vi "Create Value - Known Type.vi"(5 "JSON Compatible Type":T1=enum."Unknown", 7 "JSON Type":T2=enum."Unknown", 8 "error in (no error)":errorcluster, 10 "Value":variant) -> (0 "error out":errorcluster, 3 "JSON Tree":variant)   [LabVIEW 2013, in "i3-json.lvlib"]
uses:
  i3-json.lvlib
  JSON Types/JSON Type.ctl
  JSON Types/JSON Compatible Type.ctl
  JSON Types/JSON Variant Attribute.ctl
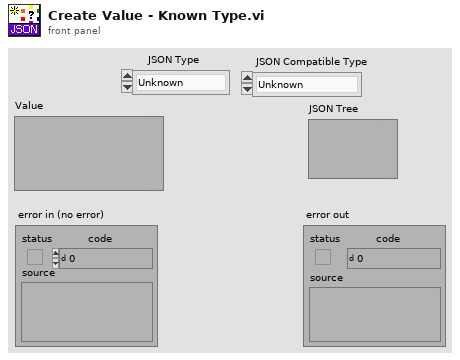
[diagram p1: front panel]
types:
  T1 = typedef "i3-json.lvlib/JSON Compatible Type.ctl" = enum16{"1D Double Array", "1D String Array", "1D Boolean Array", "Unknown"}
  T2 = typedef "i3-json.lvlib/JSON Type.ctl" = enum8{"JSON Compatible", "JSON Array", "JSON Object", "JSON Null", "Double", "String", "Boolean", "Unknown", "Data JSON string"}
  T3 = typedef "i3-json.lvlib/JSON Variant Attribute.ctl" = string
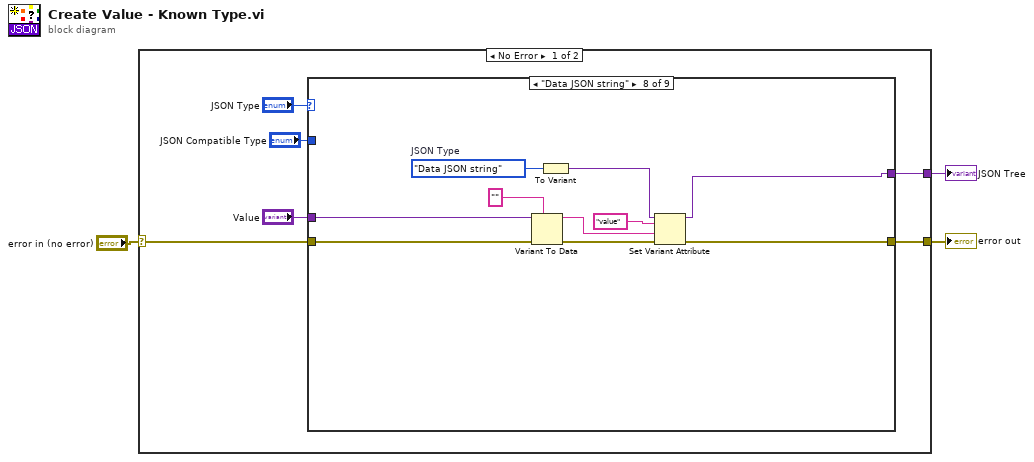
[diagram p0: block diagram]
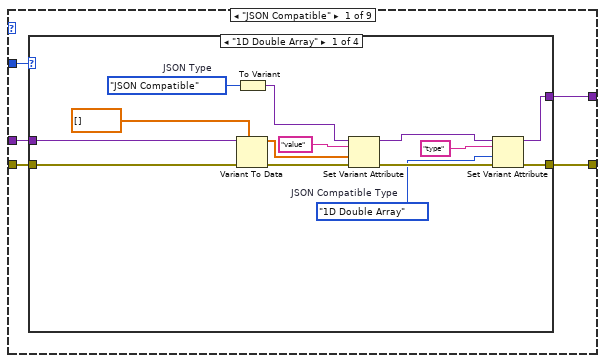
[diagram p2: hidden frame]
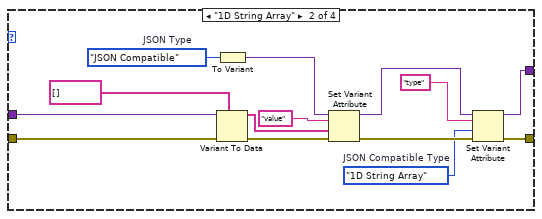
[diagram p3: hidden frame]
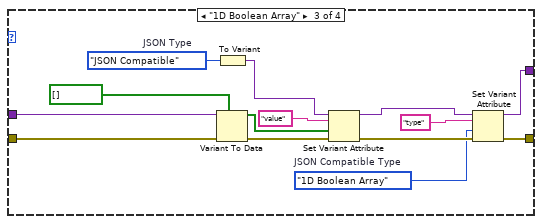
[diagram p4: hidden frame]
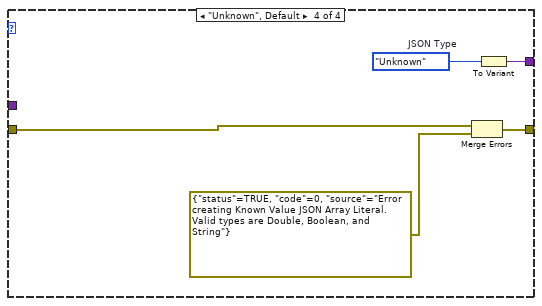
[diagram p5: hidden frame]
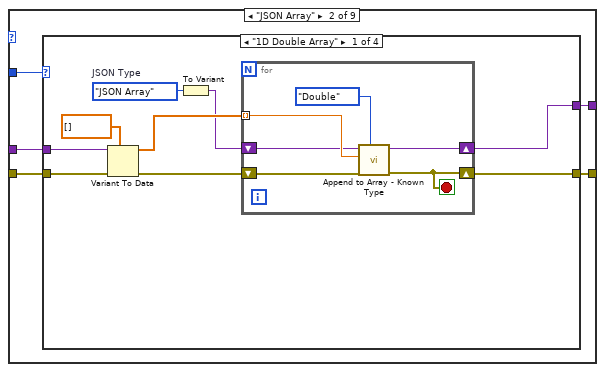
[diagram p6: hidden frame]
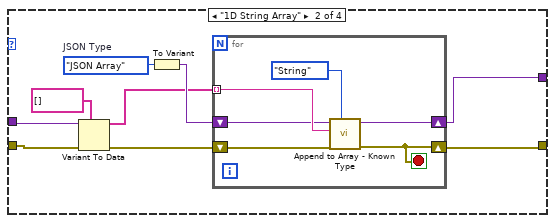
[diagram p7: hidden frame]
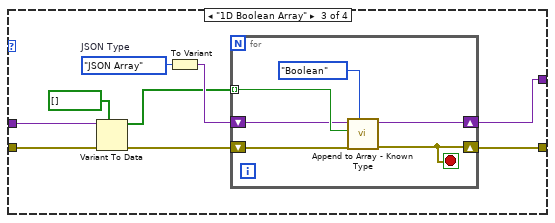
[diagram p8: hidden frame]
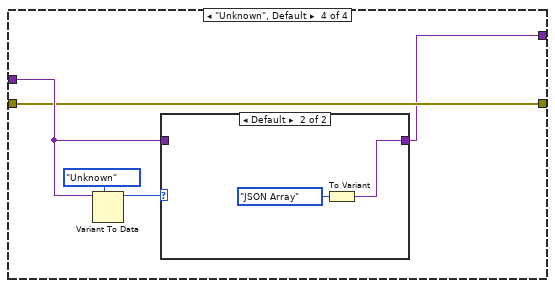
[diagram p9: hidden frame]
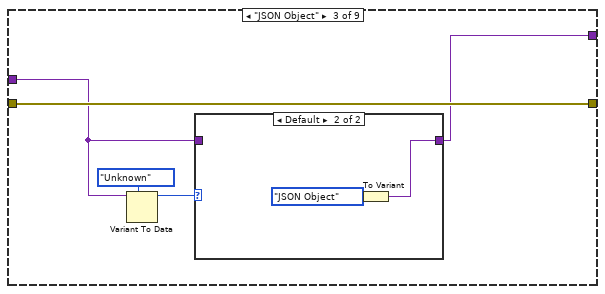
[diagram p11: hidden frame]
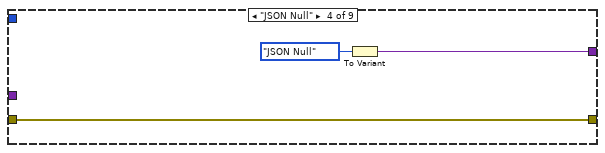
[diagram p13: hidden frame]
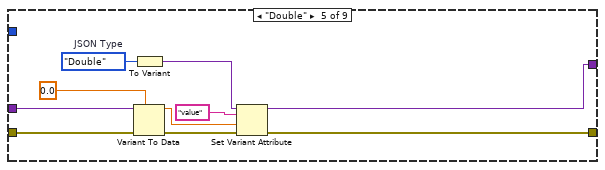
[diagram p14: hidden frame]
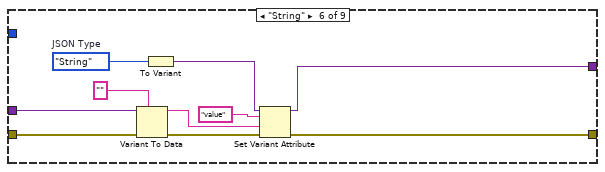
[diagram p15: hidden frame]
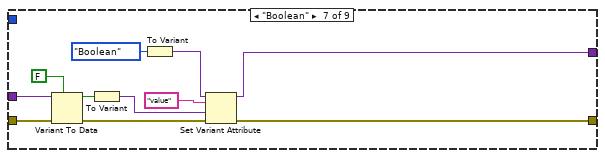
[diagram p16: hidden frame]
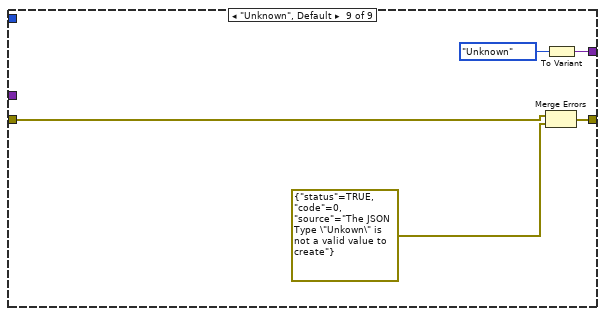
[diagram p17: hidden frame]
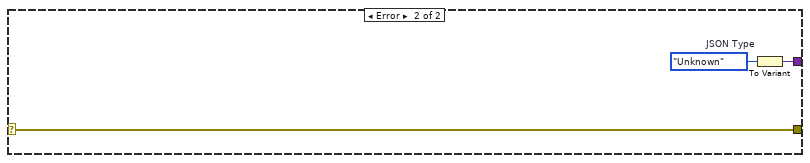
[diagram p18: hidden frame]
diagram:
  n1 = case shown="No Error" "error in (no error)" {
    selector: "error in (no error)" -> [w7 w177]
    tunnel: [w8 w177] -> w2
    tunnel: [w6 w178] -> w1
    frame No Error {
      n2 = case shown="\"Data JSON string\"" "JSON Type" {
        tunnel: [w12 w62 w124 w128 w133 w144 w152 w162 w174] -> w8
        tunnel: w7 -> [w11 w65 w124 w128 w139 w149 w159 w164 w173]
        tunnel: [w13 w66 w121 w129 w131 w145 w153 w163 w176] -> w6
        tunnel: "Value" -> [w10 w63 w122 _ w138 w148 w160 w165 _]
        tunnel: "JSON Compatible Type" -> [w14 w64 _ _ _ _ _ _ _]
        frame "JSON Compatible" {
          n3 = case shown="\"1D Double Array\"" w14 {
            tunnel: [w16 w35 w50 w59] -> w13
            tunnel: [w15 w34 w49 w61] -> w12
            tunnel: w11 -> [w19 w29 w44 w57]
            tunnel: w10 -> [w18 w32 w43 _]
            frame "1D Double Array" {
              w22 = JSON_Compatible_Type."1D Double Array"  # JSON Compatible Type
              w28 = JSON_Type."JSON Compatible"  # JSON Type
              n4 = Variant To Data(error in=w19, type=dbl[] [], Variant=w18) -> (data=w17:dbl[], error out=w20:errorcluster)
              n5 = To Variant(anything=w28) -> (Variant=w27:variant)
              n6 = Set Variant Attribute(Variant=w27, name=T3 "value" ("JSON Variant Attribute"), value=w17, error in=w20) -> (Variant out=w24:variant, error out=w26:errorcluster)  [unwired: 1 out]
              n7 = Set Variant Attribute(Variant=w24, name=T3 "type" ("JSON Variant Attribute"), value=w22, error in=w26) -> (Variant out=w16:variant, error out=w15:errorcluster)  [unwired: 1 out]
            }
            frame "1D String Array" {
              w36 = JSON_Compatible_Type."1D String Array"  # JSON Compatible Type
              w42 = JSON_Type."JSON Compatible"  # JSON Type
              n8 = Variant To Data(error in=w29, type=string[] [], Variant=w32) -> (data=w31:string[], error out=w30:errorcluster)
              n9 = To Variant(anything=w42) -> (Variant=w41:variant)
              n10 = Set Variant Attribute(Variant=w41, name=T3 "value" ("JSON Variant Attribute"), value=w31, error in=w30) -> (Variant out=w38:variant, error out=w40:errorcluster)  [unwired: 1 out]
              n11 = Set Variant Attribute(Variant=w38, name=T3 "type" ("JSON Variant Attribute"), value=w36, error in=w40) -> (Variant out=w35:variant, error out=w34:errorcluster)  [unwired: 1 out]
            }
            frame "1D Boolean Array" {
              w51 = JSON_Compatible_Type."1D Boolean Array"  # JSON Compatible Type
              w47 = JSON_Type."JSON Compatible"  # JSON Type
              n12 = Variant To Data(error in=w44, type=bool[] [], Variant=w43) -> (data=w46:bool[], error out=w45:errorcluster)
              n13 = To Variant(anything=w47) -> (Variant=w56:variant)
              n14 = Set Variant Attribute(Variant=w56, name=T3 "value" ("JSON Variant Attribute"), value=w46, error in=w45) -> (Variant out=w53:variant, error out=w55:errorcluster)  [unwired: 1 out]
              n15 = Set Variant Attribute(Variant=w53, name=T3 "type" ("JSON Variant Attribute"), value=w51, error in=w55) -> (Variant out=w50:variant, error out=w49:errorcluster)  [unwired: 1 out]
            }
            frame "Unknown", Default {
              w60 = JSON_Type."Unknown"  # JSON Type
              n16 = Merge Errors(w57, errorcluster {"status"=TRUE, "code"=0, "source"="Error creating Known Value JSON Array Literal. Valid types are Double, Boolean, and String"} ("error constant")) -> (w61:errorcluster)
              n17 = To Variant(anything=w60) -> (Variant=w59:variant)
            }
          }
        }
        frame "JSON Array" {
          n18 = case shown="\"1D Double Array\"" w64 {
            tunnel: [w67 w84 w100 w113] -> w66
            tunnel: w65 -> [w75 w83 w98 w114]
            tunnel: [w68 w85 w99 w114] -> w62
            tunnel: w63 -> [w72 w82 w97 w115]
            frame "1D Double Array" {
              w71 = JSON_Type."JSON Array"  # JSON Type
              n19 = Variant To Data(error in=w75, type=dbl[] [], Variant=w72) -> (data=w73:dbl[], error out=w69:errorcluster)
              n20 = To Variant(anything=w71) -> (Variant=w70:variant)
              n21 = for {
                shift-right: [w79] -> w67
                shift-left: w70 -> [w80]
                tunnel: w73 -> [w81] mode=indexing
                shift-right: [w76] -> w68
                shift-left: w69 -> [w77]
                stop <- w76 stop-if-true
                n22 = call "Append to Array - Known Type.vi"("JSON Type"=JSON_Type."Double", "error in (no error)"=w77, "Value"=w81, "JSON Tree in (JSON Array)"=w80) -> ("error out"=w76:errorcluster, "JSON Tree out (JSON Array)"=w79:variant)  [unwired: 6 in]
              }
            }
            frame "1D String Array" {
              w88 = JSON_Type."JSON Array"  # JSON Type
              n23 = Variant To Data(error in=w83, type=string[] [], Variant=w82) -> (data=w87:string[], error out=w90:errorcluster)
              n24 = To Variant(anything=w88) -> (Variant=w89:variant)
              n25 = for {
                shift-right: [w94] -> w84
                shift-left: w89 -> [w95]
                tunnel: w87 -> [w96] mode=indexing
                shift-right: [w91] -> w85
                shift-left: w90 -> [w92]
                stop <- w91 stop-if-true
                n26 = call "Append to Array - Known Type.vi"("JSON Type"=JSON_Type."String", "error in (no error)"=w92, "Value"=w96, "JSON Tree in (JSON Array)"=w95) -> ("error out"=w91:errorcluster, "JSON Tree out (JSON Array)"=w94:variant)  [unwired: 6 in]
              }
            }
            frame "1D Boolean Array" {
              w103 = JSON_Type."JSON Array"  # JSON Type
              n27 = Variant To Data(error in=w98, type=bool[] [], Variant=w97) -> (data=w102:bool[], error out=w105:errorcluster)
              n28 = To Variant(anything=w103) -> (Variant=w104:variant)
              n29 = for {
                shift-right: [w109] -> w100
                shift-left: w104 -> [w110]
                tunnel: w102 -> [w111] mode=indexing
                shift-right: [w106] -> w99
                shift-left: w105 -> [w107]
                stop <- w106 stop-if-true
                n30 = call "Append to Array - Known Type.vi"("JSON Type"=JSON_Type."Boolean", "error in (no error)"=w107, "Value"=w111, "JSON Tree in (JSON Array)"=w110) -> ("error out"=w106:errorcluster, "JSON Tree out (JSON Array)"=w109:variant)  [unwired: 6 in]
              }
            }
            frame "Unknown", Default {
              n31 = Variant To Data(type=JSON_Type."Unknown" ("JSON Type"), Variant=w115) -> (data=w112:T2)  [unwired: 1 in, 1 out]
              n32 = case shown="Default" w112 {
                tunnel: w115 -> [w117 _]
                tunnel: [w117 w118] -> w113
                frame "JSON Array" {
                }
                frame Default {
                  n33 = To Variant(anything=JSON_Type."JSON Array" ("JSON Type")) -> (Variant=w118:variant)
                }
              }
            }
          }
        }
        frame "JSON Object" {
          n34 = Variant To Data(type=JSON_Type."Unknown" ("JSON Type"), Variant=w122) -> (data=w120:T2)  [unwired: 1 in, 1 out]
          n35 = case shown="Default" w120 {
            tunnel: w122 -> [w125 _]
            tunnel: [w125 w126] -> w121
            frame "JSON Object" {
            }
            frame Default {
              n36 = To Variant(anything=JSON_Type."JSON Object" ("JSON Type")) -> (Variant=w126:variant)
            }
          }
        }
        frame "JSON Null" {
          n37 = To Variant(anything=JSON_Type."JSON Null" ("JSON Type")) -> (Variant=w129:variant)
        }
        frame "Double" {
          w137 = JSON_Type."Double"  # JSON Type
          n38 = Variant To Data(error in=w139, type=0.0 ("Numeric"), Variant=w138) -> (data=w132:dbl, error out=w134:errorcluster)
          n39 = To Variant(anything=w137) -> (Variant=w136:variant)
          n40 = Set Variant Attribute(Variant=w136, name=T3 "value" ("JSON Variant Attribute"), value=w132, error in=w134) -> (Variant out=w131:variant, error out=w133:errorcluster)  [unwired: 1 out]
        }
        frame "String" {
          w141 = JSON_Type."String"  # JSON Type
          n41 = Variant To Data(error in=w149, type="" ("String"), Variant=w148) -> (data=w142:string, error out=w143:errorcluster)
          n42 = To Variant(anything=w141) -> (Variant=w147:variant)
          n43 = Set Variant Attribute(Variant=w147, name=T3 "value" ("JSON Variant Attribute"), value=w142, error in=w143) -> (Variant out=w145:variant, error out=w144:errorcluster)  [unwired: 1 out]
        }
        frame "Boolean" {
          n44 = Variant To Data(error in=w159, type=FALSE ("data"), Variant=w160) -> (data=w154:bool, error out=w151:errorcluster)
          n45 = To Variant(anything=w154) -> (Variant=w155:variant)
          n46 = To Variant(anything=JSON_Type."Boolean" ("JSON Type")) -> (Variant=w157:variant)
          n47 = Set Variant Attribute(Variant=w157, name=T3 "value" ("JSON Variant Attribute"), value=w155, error in=w151) -> (Variant out=w153:variant, error out=w152:errorcluster)  [unwired: 1 out]
        }
        frame "Data JSON string" {
          w166 = JSON_Type."Data JSON string"  # JSON Type
          n48 = Variant To Data(error in=w164, type="" ("String"), Variant=w165) -> (data=w167:string, error out=w168:errorcluster)
          n49 = To Variant(anything=w166) -> (Variant=w170:variant)
          n50 = Set Variant Attribute(Variant=w170, name=T3 "value" ("JSON Variant Attribute"), value=w167, error in=w168) -> (Variant out=w163:variant, error out=w162:errorcluster)  [unwired: 1 out]
        }
        frame "Unknown", Default {
          n51 = Merge Errors(w173, errorcluster {"status"=TRUE, "code"=0, "source"="The JSON Type \"Unkown\" is not a valid value to create"} ("error out")) -> (w174:errorcluster)
          n52 = To Variant(anything=JSON_Type."Unknown" ("JSON Type")) -> (Variant=w176:variant)
        }
      }
    }
    frame Error {
      w179 = JSON_Type."Unknown"  # JSON Type
      n53 = To Variant(anything=w179) -> (Variant=w178:variant)
    }
  }
  "JSON Tree" <- w1
  "error out" <- w2
